vi "Create from SSH.vi"(8 "Error In":errorcluster, 11 "SSH":refnum<class "SSH.lvclass">) -> (0 "Error Out":errorcluster, 3 "Identity":refnum<class "Agent Identity.lvclass">)   [LabVIEW 2021, in "Field_RnD_Services_LIBSSH2_Toolkit.lvlib" / "Agent Identity.lvclass"]
doc: "Creates a new Agent Identity object fomr a SSH context."
uses:
  220524-VNA RP FLAT.llb/Agent Identity.lvclass
  220524-VNA RP FLAT.llb/SSH.lvclass
  220524-VNA RP FLAT.llb/Agent Identity.lvclass/Agent Identity.ctl
  220524-VNA RP FLAT.llb/Field_RnD_Services_LIBSSH2_Toolkit.lvlib
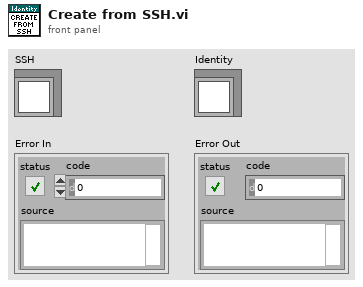
[diagram p1: front panel]
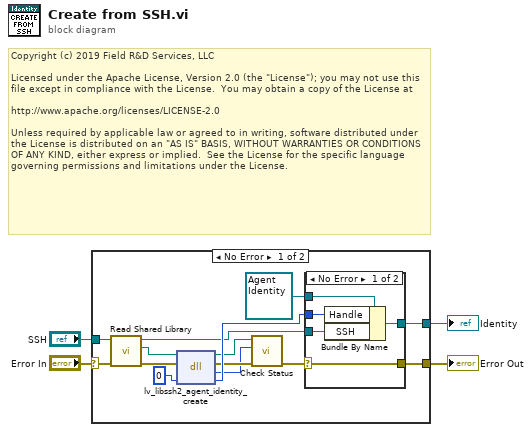
[diagram p0: block diagram]
diagram:
  # "Copyright (c) 2019 Field R&D Services, LLC\n\nLicensed under the Apache License, Version 2.0 (the \"License\"); you may not use this file except in compliance with the License.  You may obtain a copy of the License at\n\nhttp://www.apache.org/licenses/LICENSE-2.0\n\nUnless required by applicable law or agreed to in writing, software distributed under the License is distributed on an \"AS IS\" BASIS, WITHOUT WARRANTIES OR CONDITIONS OF ANY KIND, either express or implied.  See the License for the specific language governing permissions and limitations under the License."
  n1 = case shown="No Error" "Error In" {
    selector: "Error In" -> [w6 w26]
    tunnel: [w9 w26] -> w3
    tunnel: "SSH" -> [w7 _]
    tunnel: [w18 _] -> w1
    frame No Error {
      n2 = call "Read Shared Library.vi"("Error In"=w6, "SSH In"=w7) -> ("Error Out"=w17:errorcluster, "libssh2lv Shared Library"=w16:path, "SSH Out"=w8:refnum<class "SSH.lvclass">)  [unwired: 7 in]
      n3 = dll-call lib="libssh2lv.*" fn="lv_libssh2_agent_identity_create"(path in=w16, error in=w17, "handle"=u64 0) -> (path out=w11:path, error out=w13:errorcluster, "status"=w12:i32, "handle"=w14:u64)  [unwired: 1 in]
      n4 = call "Check Status.vi"("Error In"=w13, "Status"=w12, "libssh2lv Shared Library In"=w11) -> ("Error Out"=w10:errorcluster)  [unwired: 7 in, 1 out]
      n5 = case shown="No Error" w10 {
        selector: w10 -> [w22 w25]
        tunnel: [w19 w24] -> w18
        tunnel: w14 -> [w23 _]
        tunnel: [w22 w25] -> w9
        tunnel: w8 -> [w21 _]
        tunnel: refnum<class "Agent Identity.lvclass"> refnum ("Toolkit.lvlib:Agent Identity.lvclass") -> [w20 w24]
        frame No Error {
          n6 = Bundle By Name(cluster=w20, "Handle"=w23, "SSH"=w21) -> (w19:refnum<class "Agent Identity.lvclass">)
        }
        frame Error {
        }
      }
    }
    frame Error {
    }
  }
  "Error Out" <- w3
  "Identity" <- w1
